vi "Microscope ID global.vi"() -> ()   [LabVIEW 2011]
panel:
  in  "Microscope ID":string="h-nu"
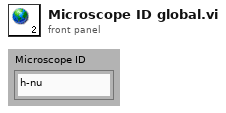
[diagram p1: front panel]
diagram:
